vi "Fit.vi"() -> ()   [LabVIEW 2011]
panel:
  in  "From Counts":string="c1+c2+c3+c4"
  out "Origin.IOApplication":refnum<k7>
  in  "stop":bool
  in  "Fit":bool
  in  "Fit Data":string(combo)="data file"
  in  "OriginLab Visible?":i32(ring) items=["MAINWND_HIDE"=0, "MAINWND_SHOW"=1, "MAINWND_SHOWMINIMIZED"=2, "MAINWND_SHOWMAXIMIZED"=3, "MAINWND_SHOW_BRING_TO_FRONT"=100]
  out "String":string
  in  "Fitting Function":string(combo)="sine"
  out "Fit":cluster{"data":dbl[], "data":dbl[]}[](graph)
  out "Peak Height":dbl
  out "Peak Width":dbl
  out "Peak Center":dbl format="%#_9g"
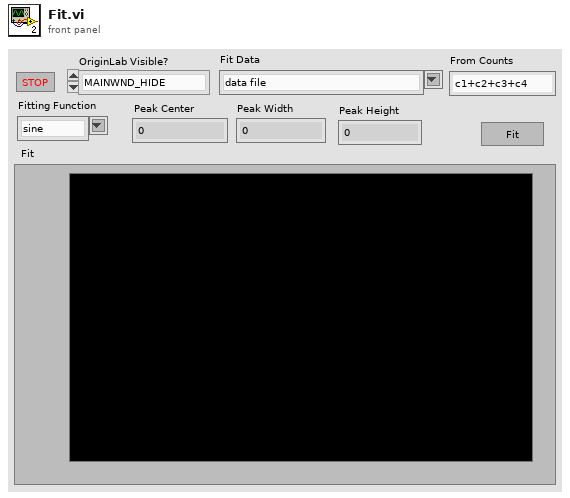
[diagram p1: front panel]
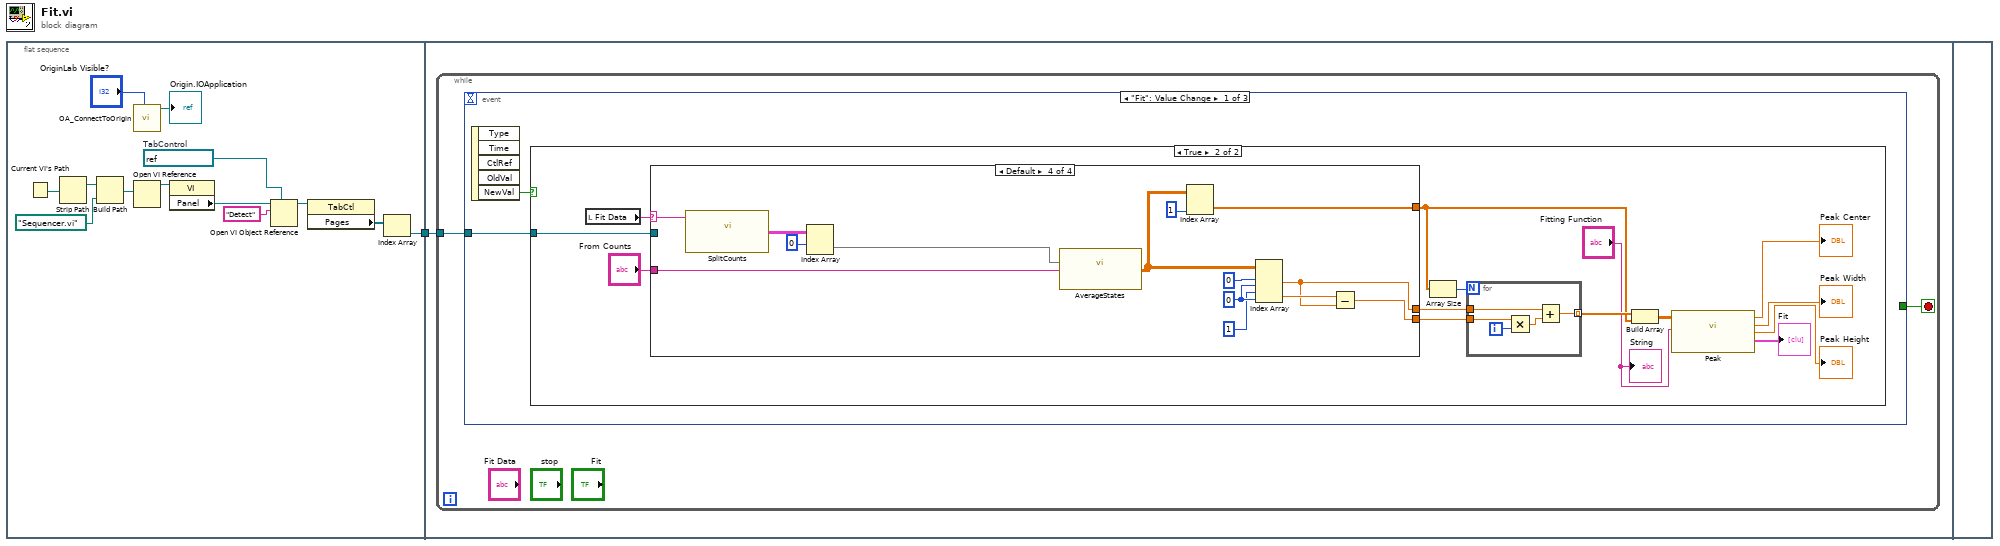
[diagram p0: block diagram]
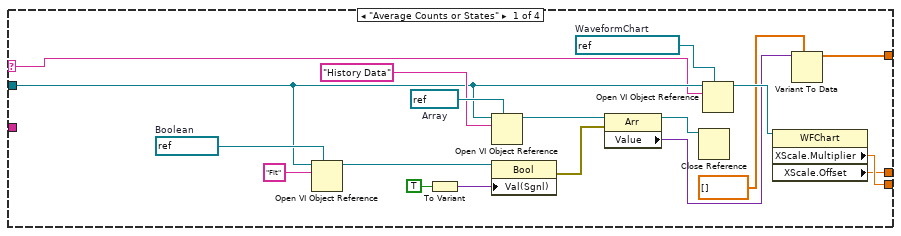
[diagram p3: hidden frame]
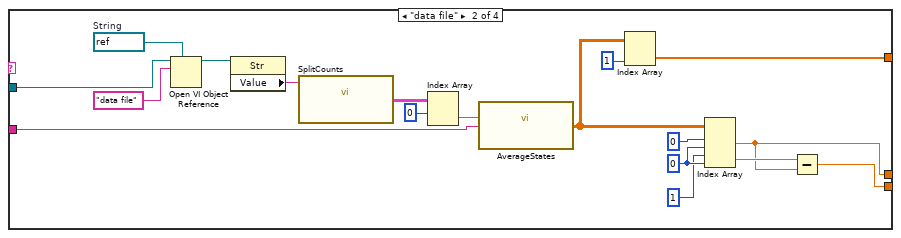
[diagram p4: hidden frame]
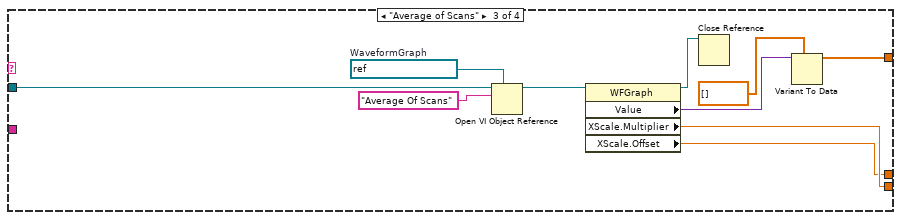
[diagram p5: hidden frame]
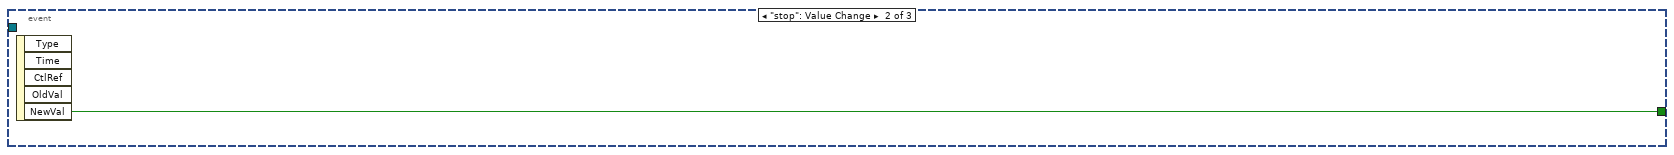
[diagram p6: hidden frame]
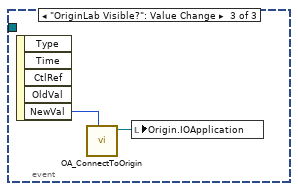
[diagram p7: hidden frame]
diagram:
  n1 = flat-sequence {
    tunnel: [w8] -> w1
    tunnel: w1 -> [w15]
    frame #0 {
      w11 = refnum<vi> refnum  # TabControl
      n2 = Current VI's Path() -> (path=w5:path)
      n3 = Strip Path(path=w5) -> (stripped path=w4:path)  [unwired: 1 out]
      n4 = Build Path(base path=w4, name or relative path=path "Sequencer.vi" ("vi path")) -> (appended path=w2:path)
      n5 = call <userlib>:"OA_ConnectToOrigin.vi"("Visible"="OriginLab Visible?") -> ("Origin.IOApplication"=→"Origin.IOApplication":refnum<k7>)  [unwired: 7 in, 1 out]
      n6 = Open VI Reference(vi path=w2) -> (vi reference=w10:refnum<vi>)  [unwired: 5 in, 1 out]
      n7 = property class="VI"(reference=w10) -> ("Panel"=w14:refnum<vi>)  [unwired: 1 in, 2 out]
      n8 = Open VI Object Reference(7:w11, 10:"Detect" ("name/order"), 11:w14) -> (3:w13:refnum<vi>)  [unwired: 1 in, 1 out]
      n9 = property class="TabCtl"(reference=w13) -> ("Pages"=w12:refnum<vi>[])  [unwired: 1 in, 2 out]
      n10 = Index Array(array=w12) -> (element=w8:refnum<vi>)  [unwired: 1 in]
    }
    frame #1 {
      n11 = while {
        tunnel: w15 -> [w17]
        stop <- w16 stop-if-true
        n12 = event shown="[0] \"Fit\": Value Change" {
          selector: _ -> [_ _ _]
          dyn-events: _ -> [_ _ _]
          timeout: _ -> [_ _ _]
          tunnel: w17 -> [w19 _ _]
          tunnel: [_ w100 _] -> w16
          event "Fit": Value Change {
            n13 = event-data() -> ("NewVal"=w18:bool)  [unwired: 1 in, 4 out]
            n14 = case shown="True" w18 {
              tunnel: w19 -> [_ w33]
              frame False {
              }
              frame True {
                n15 = local read "Fit Data"() -> (w21:string)
                n16 = case shown="Default" w21 {
                  selector: w21 -> [w39 _ _ w89]
                  tunnel: w33 -> [w49 w75 w85 _]
                  tunnel: [w52 w61 w82 w92] -> w28
                  tunnel: [w51 w62 w81 w93] -> w27
                  tunnel: [w41 w63 w78 w97] -> w22
                  tunnel: "From Counts" -> [_ w59 _ w87]
                  frame "Average Counts or States" {
                    w50 = refnum<vi> refnum  # Boolean
                    w54 = refnum<vi> refnum  # WaveformChart
                    w57 = refnum<vi> refnum  # Array
                    n17 = Open VI Object Reference(7:w50, 10:"Fit" ("name/order"), 11:w49) -> (3:w47:refnum<vi>)  [unwired: 1 in, 1 out]
                    n18 = To Variant(anything=TRUE) -> (Variant=w45:variant)
                    n19 = Open VI Object Reference(7:w57, 10:"History Data" ("name/order"), 11:w49) -> (3:w56:refnum<vi>)  [unwired: 1 in, 1 out]
                    n20 = property class="Bool"(reference=w47, "Val(Sgnl)"=w45) -> (error out=w44:errorcluster)  [unwired: 1 in, 1 out]
                    n21 = property class="Arr"(reference=w56, error in=w44) -> (reference out=w40:refnum<vi>, "Value"=w43:variant)  [unwired: 1 out]
                    n22 = Close Reference(reference=w40) -> ()  [unwired: 1 in, 1 out]
                    n23 = Open VI Object Reference(7:w54, 10:w39, 11:w49) -> (3:w53:refnum<vi>)  [unwired: 1 in, 1 out]
                    n24 = property class="WFChart"(reference=w53) -> ("XScale.Multiplier"=w52:dbl, "XScale.Offset"=w51:dbl)  [unwired: 1 in, 2 out]
                    n25 = Variant To Data(type=dbl[] [], Variant=w43) -> (data=w41:dbl[])  [unwired: 1 in, 1 out]
                  }
                  frame "data file" {
                    w69 = 0 ("disabled index (col)")
                    w72 = refnum<vi> refnum  # String
                    n26 = Open VI Object Reference(7:w72, 10:"data file" ("name/order"), 11:w75) -> (3:w73:refnum<vi>)  [unwired: 1 in, 1 out]
                    n27 = property class="Str"(reference=w73) -> ("Value"=w64:string)  [unwired: 1 in, 2 out]
                    n28 = call "SplitCounts.vi"("data name"=w64) -> ("Array"=w66:cluster{dbl, i32[], i32[], i32[], i32[]}[][])  [unwired: 1 in]
                    n29 = Index Array(array=w66, index (row)=0) -> (element=w60:cluster{dbl, i32[], i32[], i32[], i32[]}[])  [unwired: 1 in]
                    n30 = call "AverageStates.vi"("From Counts"=w59, "Counts"=w60) -> ("Values"=w58:dbl[][])  [unwired: 2 in]
                    n31 = Index Array(array=w58, index (col)=1 ("disabled index (col)")) -> (element=w63:dbl[])  [unwired: 1 in]
                    n32 = Index Array(array=w58, index (row) #1=0 ("index (row)"), index (col) #1=w69, index (row) #2=1 ("disabled index (row)"), index (col) #2=w69) -> (element #1=w62:dbl, element #2=w67:dbl)
                    n33 = Subtract(x=w67, y=w62) -> (x-y=w61:dbl)
                  }
                  frame "Average of Scans" {
                    w84 = refnum<vi> refnum  # WaveformGraph
                    n34 = Open VI Object Reference(7:w84, 10:"Average Of Scans" ("name/order"), 11:w85) -> (3:w83:refnum<vi>)  [unwired: 1 in, 1 out]
                    n35 = property class="WFGraph"(reference=w83) -> (reference out=w77:refnum<vi>, "Value"=w79:variant, "XScale.Multiplier"=w82:dbl, "XScale.Offset"=w81:dbl)  [unwired: 1 in, 1 out]
                    n36 = Close Reference(reference=w77) -> ()  [unwired: 1 in, 1 out]
                    n37 = Variant To Data(type=dbl[] [], Variant=w79) -> (data=w78:dbl[])  [unwired: 1 in, 1 out]
                  }
                  frame Default {
                    w96 = 0 ("disabled index (col)")
                    n38 = call "SplitCounts.vi"("data name"=w89) -> ("Array"=w91:cluster{dbl, i32[], i32[], i32[], i32[]}[][])  [unwired: 1 in]
                    n39 = Index Array(array=w91, index (row)=0) -> (element=w88:cluster{dbl, i32[], i32[], i32[], i32[]}[])  [unwired: 1 in]
                    n40 = call "AverageStates.vi"("From Counts"=w87, "Counts"=w88) -> ("Values"=w86:dbl[][])  [unwired: 2 in]
                    n41 = Index Array(array=w86, index (col)=1 ("disabled index (col)")) -> (element=w97:dbl[])  [unwired: 1 in]
                    n42 = Index Array(array=w86, index (row) #1=0 ("index (row)"), index (col) #1=w96, index (row) #2=1 ("disabled index (row)"), index (col) #2=w96) -> (element #1=w93:dbl, element #2=w94:dbl)
                    n43 = Subtract(x=w94, y=w93) -> (x-y=w92:dbl)
                  }
                }
                n44 = Array Size(array=w22) -> (size(s)=w24:i32)
                n45 = for {
                  N: w24 -> [_]
                  tunnel: w28 -> [w37]
                  tunnel: w27 -> [w35]
                  tunnel: [w34] -> w26 mode=indexing
                  i -> [w38]
                  n46 = Multiply(x=w37, y=w38) -> (x*y=w36:dbl)
                  n47 = Add(x=w35, y=w36) -> (x+y=w34:dbl)
                }
                n48 = Build Array(w26, w22) -> (w25:dbl[][])
                n49 = call "Peak.vi"("2d Data"=w25, "Fitting Function"="Fitting Function") -> ("Peak Center"=→"Peak Center":dbl, "Peak Width"=→"Peak Width":dbl, "Peak Height"=→"Peak Height":dbl, "Fit"=→"Fit":cluster{"data":dbl[], "data":dbl[]}[])  [unwired: 1 in]
                "String" <- "Fitting Function"
              }
            }
          }
          event "stop": Value Change {
            n50 = event-data() -> ("NewVal"=w100:bool)  [unwired: 1 in, 4 out]
          }
          event "OriginLab Visible?": Value Change {
            n51 = event-data() -> ("NewVal"=w102:i32)  [unwired: 1 in, 4 out]
            n52 = call <userlib>:"OA_ConnectToOrigin.vi"("Visible"=w102) -> ("Origin.IOApplication"=w101:refnum<k7>)  [unwired: 7 in, 1 out]
            n53 = local write "Origin.IOApplication"(w101) -> ()
          }
        }
      }
    }
    frame #2 {
    }
  }
